vi "Example All Data.vi"() -> ()   [LabVIEW 2010]
uses:
  C:/tf/play/labview/Tinkerforge.dll
  Tinkerforge.dll
panel:
  out "calibration status":u8
  out "temperature (°C)":i16
  out "gravity vector (m/s²)":sgl[](array[numeric])
  out "linear acceleration (m/s²)":sgl[](array[numeric])
  out "euler angle (°)":sgl[](array[numeric])
  out "angular velocity (°/s)":sgl[](array[numeric])
  out "magnetic field (µT)":sgl[](array[numeric])
  out "quaternion":sgl[](array[numeric])
  out "acceleration (m/s²)":sgl[](array[numeric]) format="%.2f"
  in  "stop":bool
  in  "uid":string="6wVE7W"
  in  "port":i32=4223
  in  "host":string="localhost"
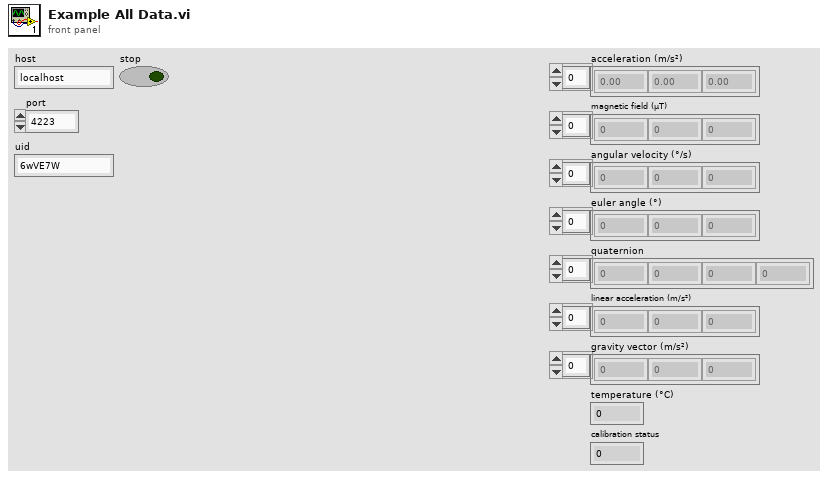
[diagram p1: front panel]
types:
  T1 = cluster{"acceleration":i16[], "magneticField":i16[], "angularVelocity":i16[], "eulerAngle":i16[], "quaternion":i16[], "linearAcceleration":i16[], "gravityVector":i16[], "temperature":i16, "calibrationStatus":u8}
  T2 = cluster{"acceleration[0]":i16, "acceleration[1]":i16, "acceleration[2]":i16, "acceleration[3]":i16, "acceleration[4]":i16, "acceleration[5]":i16, "acceleration[6]":i16, "acceleration[7]":i16, "acceleration[8]":i16}
  T3 = cluster{"magneticField[0]":i16, "magneticField[1]":i16, "magneticField[2]":i16, "magneticField[3]":i16, "magneticField[4]":i16, "magneticField[5]":i16, "magneticField[6]":i16, "magneticField[7]":i16, "magneticField[8]":i16}
  T4 = cluster{"angularVelocity[0]":i16, "angularVelocity[1]":i16, "angularVelocity[2]":i16, "angularVelocity[3]":i16, "angularVelocity[4]":i16, "angularVelocity[5]":i16, "angularVelocity[6]":i16, "angularVelocity[7]":i16, "angularVelocity[8]":i16}
  T5 = cluster{"eulerAngle[0]":i16, "eulerAngle[1]":i16, "eulerAngle[2]":i16, "eulerAngle[3]":i16, "eulerAngle[4]":i16, "eulerAngle[5]":i16, "eulerAngle[6]":i16, "eulerAngle[7]":i16, "eulerAngle[8]":i16}
  T6 = cluster{"quaternion[0]":i16, "quaternion[1]":i16, "quaternion[2]":i16, "quaternion[3]":i16, "quaternion[4]":i16, "quaternion[5]":i16, "quaternion[6]":i16, "quaternion[7]":i16, "quaternion[8]":i16}
  T7 = cluster{"linearAcceleration[0]":i16, "linearAcceleration[1]":i16, "linearAcceleration[2]":i16, "linearAcceleration[3]":i16, "linearAcceleration[4]":i16, "linearAcceleration[5]":i16, "linearAcceleration[6]":i16, "linearAcceleration[7]":i16, "linearAcceleration[8]":i16}
  T8 = cluster{"gravityVector[0]":i16, "gravityVector[1]":i16, "gravityVector[2]":i16, "gravityVector[3]":i16, "gravityVector[4]":i16, "gravityVector[5]":i16, "gravityVector[6]":i16, "gravityVector[7]":i16, "gravityVector[8]":i16}
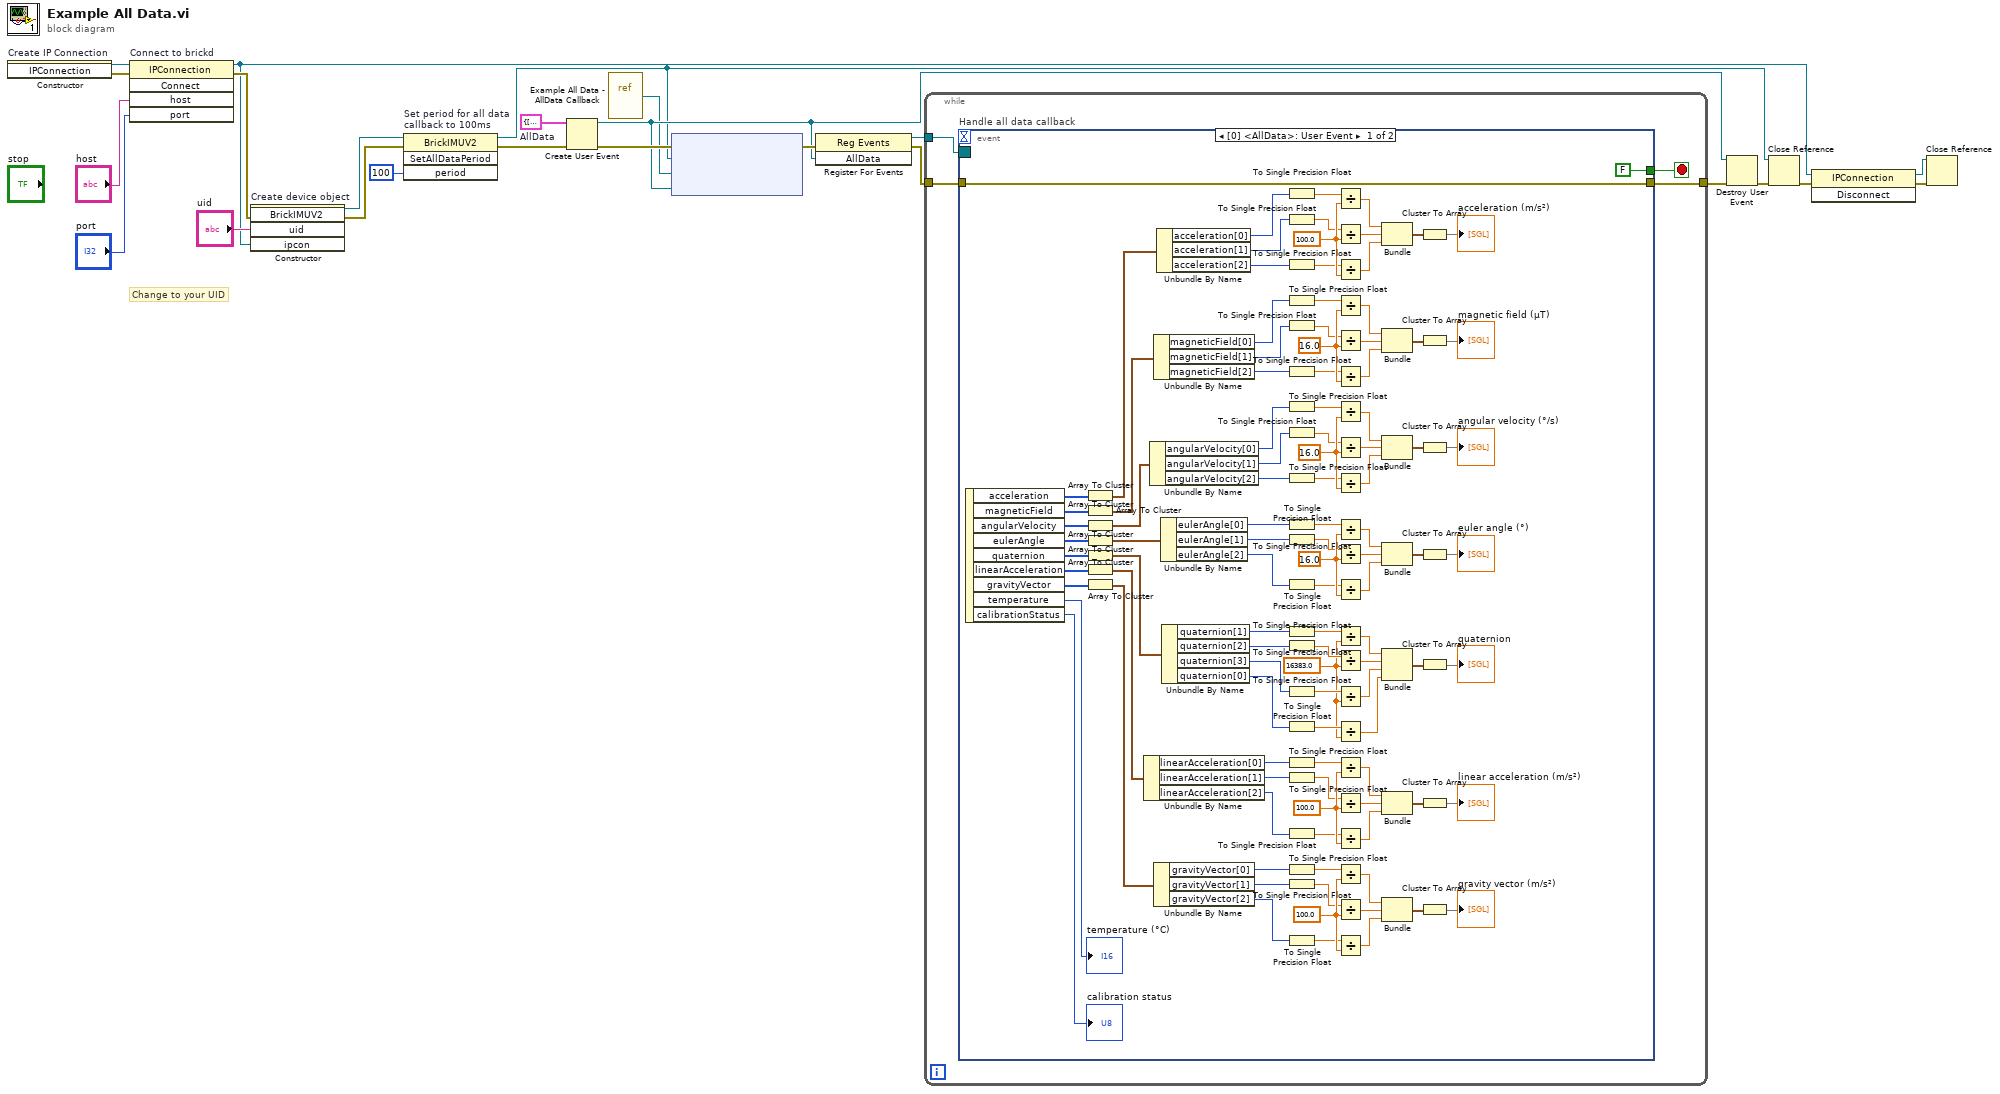
[diagram p0: block diagram]
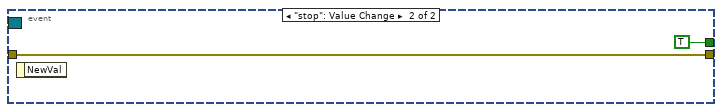
[diagram p2: hidden frame]
diagram:
  w8 = T1 {"acceleration"=[], "magneticField"=[], "angularVelocity"=[], "eulerAngle"=[], "quaternion"=[], "linearAcceleration"=[], "gravityVector"=[], "temperature"=0, "calibrationStatus"=0}  # AllData
  # "Change to your UID"
  n1 = constructor on="Create IP Connection" class="IPConnection"() -> (reference out=w24:refnum<k24>, error out=w2:errorcluster)  [unwired: 3 in, 1 out]
  n2 = invoke on="Connect to brickd" class="IPConnection" method="Connect"(reference=w24, error in=w2, "host"="host", "port"="port") -> (reference out=w17:refnum<k24>, error out=w20:errorcluster)  [unwired: 1 in, 3 out]
  n3 = constructor on="Create device object" class="BrickIMUV2"(error in=w20, "uid"="uid", "ipcon"=w17) -> (reference out=w5:refnum<k24>, error out=w7:errorcluster)  [unwired: 2 in, 3 out]
  n4 = invoke on="Set period for all data\ncallback to 100ms" class="BrickIMUV2" method="SetAllDataPeriod"(reference=w5, error in=w7, "period"=i64 100) -> (reference out=w4:refnum<k24>, error out=w6:errorcluster)  [unwired: 1 in, 2 out]
  n5 = Create User Event(user event datatype=w8, error in=w6) -> (user event=w10:refnum<user-event>, error out=w15:errorcluster)
  n6 = vi-ref "Example All Data - AllData Callback.vi"() -> ("vi reference"=w1:refnum<vi>)
  n7 = node ("Register Event Callback")(w15, w4, w1, w10) -> (w14:errorcluster)  [unwired: 1 in, 1 out]
  n8 = register-events(error in=w14, w10) -> (reference out=w13:refnum<event-registration>, error out=w11:errorcluster)  [unwired: 1 in]
  n9 = while {
    tunnel: w13 -> [w28]
    tunnel: [w27] -> w12
    tunnel: w11 -> [w26]
    stop <- w25 stop-if-true
    n10 = event "Handle all data callback" shown="[0] <AllData>: User Event" {
      selector: w28 -> [_ _]
      dyn-events: _ -> [_ _]
      timeout: _ -> [_ _]
      tunnel: [w133 w134] -> w27
      tunnel: w26 -> [w133 w134]
      tunnel: [FALSE TRUE] -> w25
      event User Event {
        w37 = sgl 100.0 ("y")
        w51 = sgl 100.0 ("y")
        w65 = sgl 16.0 ("y")
        w79 = sgl 16.0 ("y")
        w93 = sgl 16.0 ("y")
        w102 = sgl 16383.0 ("y")
        w122 = sgl 100.0 ("y")
        n11 = event-data() -> ("acceleration"=w131:i16[], "magneticField"=w88:i16[], "angularVelocity"=w74:i16[], "eulerAngle"=w59:i16[], "quaternion"=w106:i16[], "linearAcceleration"=w46:i16[], "gravityVector"=w32:i16[], "temperature"=→"temperature (°C)":i16, "calibrationStatus"=→"calibration status":u8)  [unwired: 1 in]
        n12 = Array To Cluster(array=w131) -> (cluster=w130:T2)
        n13 = Array To Cluster(array=w88) -> (cluster=w100:T3)
        n14 = Array To Cluster(array=w74) -> (cluster=w86:T4)
        n15 = Array To Cluster(array=w59) -> (cluster=w72:T5)
        n16 = Array To Cluster(array=w106) -> (cluster=w117:T6)
        n17 = Array To Cluster(array=w46) -> (cluster=w58:T7)
        n18 = Array To Cluster(array=w32) -> (cluster=w44:T8)
        n19 = Unbundle By Name(w58) -> ("linearAcceleration[0]"=w53:i16, "linearAcceleration[1]"=w50:i16, "linearAcceleration[2]"=w49:i16)
        n20 = Unbundle By Name(w86) -> ("angularVelocity[0]"=w81:i16, "angularVelocity[1]"=w78:i16, "angularVelocity[2]"=w77:i16)
        n21 = Unbundle By Name(w100) -> ("magneticField[0]"=w95:i16, "magneticField[1]"=w92:i16, "magneticField[2]"=w91:i16)
        n22 = Unbundle By Name(w44) -> ("gravityVector[0]"=w39:i16, "gravityVector[1]"=w36:i16, "gravityVector[2]"=w35:i16)
        n23 = Unbundle By Name(w130) -> ("acceleration[0]"=w124:i16, "acceleration[1]"=w121:i16, "acceleration[2]"=w120:i16)
        n24 = Unbundle By Name(w72) -> ("eulerAngle[0]"=w67:i16, "eulerAngle[1]"=w64:i16, "eulerAngle[2]"=w63:i16)
        n25 = Unbundle By Name(w117) -> ("quaternion[1]"=w112:i16, "quaternion[2]"=w110:i16, "quaternion[3]"=w109:i16, "quaternion[0]"=w103:i16)
        n26 = To Single Precision Float(number=w124) -> (single precision float=w123:sgl)
        n27 = To Single Precision Float(number=w121) -> (single precision float=w119:sgl)
        n28 = To Single Precision Float(number=w120) -> (single precision float=w118:sgl)
        n29 = To Single Precision Float(number=w95) -> (single precision float=w94:sgl)
        n30 = To Single Precision Float(number=w92) -> (single precision float=w90:sgl)
        n31 = To Single Precision Float(number=w91) -> (single precision float=w89:sgl)
        n32 = To Single Precision Float(number=w81) -> (single precision float=w80:sgl)
        n33 = To Single Precision Float(number=w78) -> (single precision float=w76:sgl)
        n34 = To Single Precision Float(number=w77) -> (single precision float=w75:sgl)
        n35 = To Single Precision Float(number=w67) -> (single precision float=w66:sgl)
        n36 = To Single Precision Float(number=w64) -> (single precision float=w62:sgl)
        n37 = To Single Precision Float(number=w63) -> (single precision float=w61:sgl)
        n38 = To Single Precision Float(number=w112) -> (single precision float=w111:sgl)
        n39 = To Single Precision Float(number=w110) -> (single precision float=w108:sgl)
        n40 = To Single Precision Float(number=w109) -> (single precision float=w107:sgl)
        n41 = To Single Precision Float(number=w103) -> (single precision float=w105:sgl)
        n42 = To Single Precision Float(number=w53) -> (single precision float=w52:sgl)
        n43 = To Single Precision Float(number=w50) -> (single precision float=w48:sgl)
        n44 = To Single Precision Float(number=w49) -> (single precision float=w47:sgl)
        n45 = To Single Precision Float(number=w39) -> (single precision float=w38:sgl)
        n46 = To Single Precision Float(number=w36) -> (single precision float=w34:sgl)
        n47 = To Single Precision Float(number=w35) -> (single precision float=w33:sgl)
        n48 = Divide(x=w123, y=w122) -> (x/y=w127:sgl)
        n49 = Divide(x=w119, y=w122) -> (x/y=w126:sgl)
        n50 = Divide(x=w118, y=w122) -> (x/y=w125:sgl)
        n51 = Divide(x=w94, y=w93) -> (x/y=w98:sgl)
        n52 = Divide(x=w90, y=w93) -> (x/y=w97:sgl)
        n53 = Divide(x=w89, y=w93) -> (x/y=w96:sgl)
        n54 = Divide(x=w80, y=w79) -> (x/y=w84:sgl)
        n55 = Divide(x=w76, y=w79) -> (x/y=w83:sgl)
        n56 = Divide(x=w75, y=w79) -> (x/y=w82:sgl)
        n57 = Divide(x=w66, y=w65) -> (x/y=w70:sgl)
        n58 = Divide(x=w62, y=w65) -> (x/y=w69:sgl)
        n59 = Divide(x=w61, y=w65) -> (x/y=w68:sgl)
        n60 = Divide(x=w111, y=w102) -> (x/y=w115:sgl)
        n61 = Divide(x=w108, y=w102) -> (x/y=w114:sgl)
        n62 = Divide(x=w107, y=w102) -> (x/y=w113:sgl)
        n63 = Divide(x=w105, y=w102) -> (x/y=w104:sgl)
        n64 = Divide(x=w52, y=w51) -> (x/y=w56:sgl)
        n65 = Divide(x=w48, y=w51) -> (x/y=w55:sgl)
        n66 = Divide(x=w47, y=w51) -> (x/y=w54:sgl)
        n67 = Divide(x=w38, y=w37) -> (x/y=w42:sgl)
        n68 = Divide(x=w34, y=w37) -> (x/y=w41:sgl)
        n69 = Divide(x=w33, y=w37) -> (x/y=w40:sgl)
        n70 = Bundle(w127, w126, w125) -> (w129:cluster{sgl, sgl, sgl})  [unwired: 1 in]
        n71 = Bundle(w98, w97, w96) -> (w99:cluster{sgl, sgl, sgl})  [unwired: 1 in]
        n72 = Bundle(w84, w83, w82) -> (w85:cluster{sgl, sgl, sgl})  [unwired: 1 in]
        n73 = Bundle(w70, w69, w68) -> (w71:cluster{sgl, sgl, sgl})  [unwired: 1 in]
        n74 = Bundle(w115, w114, w113, w104) -> (w116:cluster{sgl, sgl, sgl, sgl})  [unwired: 1 in]
        n75 = Bundle(w56, w55, w54) -> (w57:cluster{sgl, sgl, sgl})  [unwired: 1 in]
        n76 = Bundle(w42, w41, w40) -> (w43:cluster{sgl, sgl, sgl})  [unwired: 1 in]
        n77 = Cluster To Array(cluster=w129) -> (array=→"acceleration (m/s²)":sgl[])
        n78 = Cluster To Array(cluster=w99) -> (array=→"magnetic field (µT)":sgl[])
        n79 = Cluster To Array(cluster=w85) -> (array=→"angular velocity (°/s)":sgl[])
        n80 = Cluster To Array(cluster=w71) -> (array=→"euler angle (°)":sgl[])
        n81 = Cluster To Array(cluster=w116) -> (array=→"quaternion":sgl[])
        n82 = Cluster To Array(cluster=w57) -> (array=→"linear acceleration (m/s²)":sgl[])
        n83 = Cluster To Array(cluster=w43) -> (array=→"gravity vector (m/s²)":sgl[])
      }
      event "stop": Value Change {
        n84 = event-data() -> ()  [unwired: 1 in, 1 out]
      }
    }
  }
  n85 = Destroy User Event(user event=w10, error in=w12) -> (error out=w9:errorcluster)
  n86 = Close Reference(reference=w4, error in (no error)=w9) -> (error out=w19:errorcluster)
  n87 = invoke class="IPConnection" method="Disconnect"(reference=w17, error in=w19) -> (reference out=w16:refnum<k24>, error out=w18:errorcluster)  [unwired: 1 in, 1 out]
  n88 = Close Reference(reference=w16, error in (no error)=w18) -> ()  [unwired: 1 out]
